vi "Lab Panel V6.00.vi"() -> ()   [LabVIEW 2017] (continued)
                            n2530 = Bundle(cluster=w4592, "amps"=w4596, "volts"=w4595, "pf"=w4594) -> (w4593:cluster{"amps":dbl, "volts":dbl, "pf":dbl})
                            n2531 = local write "ON L03-2"(w4593) -> ()
                          }
                        }
                      }
                      frame #1 {
                        n2532 = Unbundle(w4601) -> ("amps"=w4600:dbl, "volts"=w4599:dbl, "pf"=w4598:dbl)
                        n2533 = case shown="True" w4602 {
                          tunnel: w4609 -> [_ w4641]
                          tunnel: w4608 -> [_ w4648]
                          tunnel: w4607 -> [_ _]
                          tunnel: w4606 -> [_ _]
                          tunnel: w4605 -> [_ w4647]
                          tunnel: w4604 -> [_ w4646]
                          tunnel: w4603 -> [_ w4611]
                          tunnel: w4600 -> [_ w4643]
                          tunnel: w4599 -> [_ w4642]
                          tunnel: w4598 -> [_ w4640]
                          tunnel: w4597 -> [_ w4632]
                          frame False {
                          }
                          frame True {
                            n2534 = local read "TDMS LAB03-2"() -> (w4645:refnum<k34>)
                            n2535 = Build Array(w4642) -> (w4637:dbl[])
                            n2536 = Build Array(w4640) -> (w4636:dbl[])
                            n2537 = Build Array(w4647) -> (w4635:dbl[])
                            n2538 = Build Array(w4648) -> (w4634:dbl[])
                            n2539 = Build Array(w4643) -> (w4639:dbl[])
                            n2540 = Build Array(w4641) -> (w4638:dbl[])
                            n2541 = Build Array(w4646) -> (w4633:dbl[])
                            n2542 = Build Array("AMPS ON", "AMPS OFF", "VOLTS", "PF", "TEMP Live", "TEMP Neut", "CYCLE") -> (w4616:string[])
                            n2543 = Bundle By Name("Y"=w4639, "t0"=w4632) -> (w4631:waveform(dbl))  [unwired: 1 in]
                            n2544 = Bundle By Name("Y"=w4638, "t0"=w4632) -> (w4630:waveform(dbl))  [unwired: 1 in]
                            n2545 = Bundle By Name("Y"=w4637, "t0"=w4632) -> (w4629:waveform(dbl))  [unwired: 1 in]
                            n2546 = Bundle By Name("Y"=w4636, "t0"=w4632) -> (w4628:waveform(dbl))  [unwired: 1 in]
                            n2547 = Bundle By Name("Y"=w4635, "t0"=w4632) -> (w4627:waveform(dbl))  [unwired: 1 in]
                            n2548 = Bundle By Name("Y"=w4634, "t0"=w4632) -> (w4626:waveform(dbl))  [unwired: 1 in]
                            n2549 = Bundle By Name("Y"=w4633, "t0"=w4632) -> (w4625:waveform(dbl))  [unwired: 1 in]
                            n2550 = Build Array(w4631, w4630, w4629, w4628, w4627, w4626, w4625) -> (w4624:waveform(dbl)[])
                            n2551 = TDMS Write(0:w4645, 5:"TEST VALUES", 7:w4616, 9:w4624) -> (4:w4615:refnum<k34>, 6:w4614:string, 15:w4613:errorcluster)  [unwired: 2 in, 1 out]
                            n2552 = TDMS Write(0:w4615, 5:w4614, 7:"TIME", 9:w4611, 11:w4613) -> (15:w4610:errorcluster)  [unwired: 1 in, 3 out]
                            n2553 = local write "data file error"(w4610) -> ()
                          }
                        }
                      }
                    }
                  }
                }
              }
              frame #6 {
                n2554 = case shown="True" w4649 {
                  tunnel: w4653 -> [_ w4658]
                  tunnel: w4652 -> [_ w4657]
                  tunnel: w4651 -> [_ w4655]
                  tunnel: w4650 -> [_ w4654]
                  frame False {
                  }
                  frame True {
                    n2555 = local read "DISP LAB04-1"() -> (w4659:T4)
                    n2556 = local read "SIG LAB04-1"() -> (w4660:T2)
                    n2557 = local read "ON L04-1"() -> (w4656:cluster{"amps":dbl, "volts":dbl, "pf":dbl})
                    n2558 = Unbundle(w4660) -> ("AMPS"=w4666:dbl, "VOLTS"=w4664:dbl, "PF"=w4663:dbl, "Tmp Live"=w4662:dbl, "Tmp Neut"=w4665:dbl)
                    n2559 = Unbundle(w4659) -> ("CYCLE"=w4661:dbl)  [unwired: 2 out]
                    n2560 = stacked-sequence {
                      tunnel: w4666 -> [w4670 w4689]
                      tunnel: w4665 -> [_ w4688]
                      tunnel: w4664 -> [w4669 w4687]
                      tunnel: w4663 -> [w4668 w4686]
                      tunnel: w4662 -> [_ w4685]
                      tunnel: w4661 -> [_ w4684]
                      tunnel: w4658 -> [_ w4683]
                      tunnel: w4657 -> [w4671 _]
                      tunnel: w4656 -> [w4667 w4681]
                      tunnel: w4655 -> [_ w4682]
                      tunnel: w4654 -> [_ w4677]
                      frame #0 {
                        n2561 = case shown="True" w4671 {
                          tunnel: w4670 -> [_ w4676]
                          tunnel: w4669 -> [_ w4675]
                          tunnel: w4668 -> [_ w4674]
                          tunnel: w4667 -> [_ w4672]
                          frame False {
                          }
                          frame True {
                            n2562 = Bundle(cluster=w4672, "amps"=w4676, "volts"=w4675, "pf"=w4674) -> (w4673:cluster{"amps":dbl, "volts":dbl, "pf":dbl})
                            n2563 = local write "ON L04-1"(w4673) -> ()
                          }
                        }
                      }
                      frame #1 {
                        n2564 = Unbundle(w4681) -> ("amps"=w4680:dbl, "volts"=w4679:dbl, "pf"=w4678:dbl)
                        n2565 = case shown="True" w4682 {
                          tunnel: w4689 -> [_ w4721]
                          tunnel: w4688 -> [_ w4728]
                          tunnel: w4687 -> [_ _]
                          tunnel: w4686 -> [_ _]
                          tunnel: w4685 -> [_ w4727]
                          tunnel: w4684 -> [_ w4726]
                          tunnel: w4683 -> [_ w4691]
                          tunnel: w4680 -> [_ w4723]
                          tunnel: w4679 -> [_ w4722]
                          tunnel: w4678 -> [_ w4720]
                          tunnel: w4677 -> [_ w4712]
                          frame False {
                          }
                          frame True {
                            n2566 = local read "TDMS LAB04-1"() -> (w4725:refnum<k34>)
                            n2567 = Build Array(w4722) -> (w4717:dbl[])
                            n2568 = Build Array(w4720) -> (w4716:dbl[])
                            n2569 = Build Array(w4727) -> (w4715:dbl[])
                            n2570 = Build Array(w4728) -> (w4714:dbl[])
                            n2571 = Build Array(w4723) -> (w4719:dbl[])
                            n2572 = Build Array(w4721) -> (w4718:dbl[])
                            n2573 = Build Array(w4726) -> (w4713:dbl[])
                            n2574 = Build Array("AMPS ON", "AMPS OFF", "VOLTS", "PF", "TEMP Live", "TEMP Neut", "CYCLE") -> (w4696:string[])
                            n2575 = Bundle By Name("Y"=w4719, "t0"=w4712) -> (w4711:waveform(dbl))  [unwired: 1 in]
                            n2576 = Bundle By Name("Y"=w4718, "t0"=w4712) -> (w4710:waveform(dbl))  [unwired: 1 in]
                            n2577 = Bundle By Name("Y"=w4717, "t0"=w4712) -> (w4709:waveform(dbl))  [unwired: 1 in]
                            n2578 = Bundle By Name("Y"=w4716, "t0"=w4712) -> (w4708:waveform(dbl))  [unwired: 1 in]
                            n2579 = Bundle By Name("Y"=w4715, "t0"=w4712) -> (w4707:waveform(dbl))  [unwired: 1 in]
                            n2580 = Bundle By Name("Y"=w4714, "t0"=w4712) -> (w4706:waveform(dbl))  [unwired: 1 in]
                            n2581 = Bundle By Name("Y"=w4713, "t0"=w4712) -> (w4705:waveform(dbl))  [unwired: 1 in]
                            n2582 = Build Array(w4711, w4710, w4709, w4708, w4707, w4706, w4705) -> (w4704:waveform(dbl)[])
                            n2583 = TDMS Write(0:w4725, 5:"TEST VALUES", 7:w4696, 9:w4704) -> (4:w4695:refnum<k34>, 6:w4694:string, 15:w4693:errorcluster)  [unwired: 2 in, 1 out]
                            n2584 = TDMS Write(0:w4695, 5:w4694, 7:"TIME", 9:w4691, 11:w4693) -> (15:w4690:errorcluster)  [unwired: 1 in, 3 out]
                            n2585 = local write "data file error"(w4690) -> ()
                          }
                        }
                      }
                    }
                  }
                }
              }
              frame #7 {
                n2586 = case shown="True" w4729 {
                  tunnel: w4733 -> [_ w4738]
                  tunnel: w4732 -> [_ w4737]
                  tunnel: w4731 -> [_ w4735]
                  tunnel: w4730 -> [_ w4734]
                  frame False {
                  }
                  frame True {
                    n2587 = local read "DISP LAB04-2"() -> (w4739:T4)
                    n2588 = local read "SIG LAB04-2"() -> (w4740:T2)
                    n2589 = local read "ON L04-2"() -> (w4736:cluster{"amps":dbl, "volts":dbl, "pf":dbl})
                    n2590 = Unbundle(w4740) -> ("AMPS"=w4746:dbl, "VOLTS"=w4744:dbl, "PF"=w4743:dbl, "Tmp Live"=w4742:dbl, "Tmp Neut"=w4745:dbl)
                    n2591 = Unbundle(w4739) -> ("CYCLE"=w4741:dbl)  [unwired: 2 out]
                    n2592 = stacked-sequence {
                      tunnel: w4746 -> [w4750 w4769]
                      tunnel: w4745 -> [_ w4768]
                      tunnel: w4744 -> [w4749 w4767]
                      tunnel: w4743 -> [w4748 w4766]
                      tunnel: w4742 -> [_ w4765]
                      tunnel: w4741 -> [_ w4764]
                      tunnel: w4738 -> [_ w4763]
                      tunnel: w4737 -> [w4751 _]
                      tunnel: w4736 -> [w4747 w4761]
                      tunnel: w4735 -> [_ w4762]
                      tunnel: w4734 -> [_ w4757]
                      frame #0 {
                        n2593 = case shown="True" w4751 {
                          tunnel: w4750 -> [_ w4756]
                          tunnel: w4749 -> [_ w4755]
                          tunnel: w4748 -> [_ w4754]
                          tunnel: w4747 -> [_ w4752]
                          frame False {
                          }
                          frame True {
                            n2594 = Bundle(cluster=w4752, "amps"=w4756, "volts"=w4755, "pf"=w4754) -> (w4753:cluster{"amps":dbl, "volts":dbl, "pf":dbl})
                            n2595 = local write "ON L04-2"(w4753) -> ()
                          }
                        }
                      }
                      frame #1 {
                        n2596 = Unbundle(w4761) -> ("amps"=w4760:dbl, "volts"=w4759:dbl, "pf"=w4758:dbl)
                        n2597 = case shown="True" w4762 {
                          tunnel: w4769 -> [_ w4801]
                          tunnel: w4768 -> [_ w4808]
                          tunnel: w4767 -> [_ _]
                          tunnel: w4766 -> [_ _]
                          tunnel: w4765 -> [_ w4807]
                          tunnel: w4764 -> [_ w4806]
                          tunnel: w4763 -> [_ w4771]
                          tunnel: w4760 -> [_ w4803]
                          tunnel: w4759 -> [_ w4802]
                          tunnel: w4758 -> [_ w4800]
                          tunnel: w4757 -> [_ w4792]
                          frame False {
                          }
                          frame True {
                            n2598 = local read "TDMS LAB04-2"() -> (w4805:refnum<k34>)
                            n2599 = Build Array(w4802) -> (w4797:dbl[])
                            n2600 = Build Array(w4800) -> (w4796:dbl[])
                            n2601 = Build Array(w4807) -> (w4795:dbl[])
                            n2602 = Build Array(w4808) -> (w4794:dbl[])
                            n2603 = Build Array(w4803) -> (w4799:dbl[])
                            n2604 = Build Array(w4801) -> (w4798:dbl[])
                            n2605 = Build Array(w4806) -> (w4793:dbl[])
                            n2606 = Build Array("AMPS ON", "AMPS OFF", "VOLTS", "PF", "TEMP Live", "TEMP Neut", "CYCLE") -> (w4776:string[])
                            n2607 = Bundle By Name("Y"=w4799, "t0"=w4792) -> (w4791:waveform(dbl))  [unwired: 1 in]
                            n2608 = Bundle By Name("Y"=w4798, "t0"=w4792) -> (w4790:waveform(dbl))  [unwired: 1 in]
                            n2609 = Bundle By Name("Y"=w4797, "t0"=w4792) -> (w4789:waveform(dbl))  [unwired: 1 in]
                            n2610 = Bundle By Name("Y"=w4796, "t0"=w4792) -> (w4788:waveform(dbl))  [unwired: 1 in]
                            n2611 = Bundle By Name("Y"=w4795, "t0"=w4792) -> (w4787:waveform(dbl))  [unwired: 1 in]
                            n2612 = Bundle By Name("Y"=w4794, "t0"=w4792) -> (w4786:waveform(dbl))  [unwired: 1 in]
                            n2613 = Bundle By Name("Y"=w4793, "t0"=w4792) -> (w4785:waveform(dbl))  [unwired: 1 in]
                            n2614 = Build Array(w4791, w4790, w4789, w4788, w4787, w4786, w4785) -> (w4784:waveform(dbl)[])
                            n2615 = TDMS Write(0:w4805, 5:"TEST VALUES", 7:w4776, 9:w4784) -> (4:w4775:refnum<k34>, 6:w4774:string, 15:w4773:errorcluster)  [unwired: 2 in, 1 out]
                            n2616 = TDMS Write(0:w4775, 5:w4774, 7:"TIME", 9:w4771, 11:w4773) -> (15:w4770:errorcluster)  [unwired: 1 in, 3 out]
                            n2617 = local write "data file error"(w4770) -> ()
                          }
                        }
                      }
                    }
                  }
                }
              }
              frame #8 {
                n2618 = case shown="True" w4809 {
                  tunnel: w4813 -> [_ w4818]
                  tunnel: w4812 -> [_ w4817]
                  tunnel: w4811 -> [_ w4815]
                  tunnel: w4810 -> [_ w4814]
                  frame False {
                  }
                  frame True {
                    n2619 = local read "DISP LAB05-1"() -> (w4819:T4)
                    n2620 = local read "SIG LAB05-1"() -> (w4820:T2)
                    n2621 = local read "ON L05-1"() -> (w4816:cluster{"amps":dbl, "volts":dbl, "pf":dbl})
                    n2622 = Unbundle(w4820) -> ("AMPS"=w4826:dbl, "VOLTS"=w4824:dbl, "PF"=w4823:dbl, "Tmp Live"=w4822:dbl, "Tmp Neut"=w4825:dbl)
                    n2623 = Unbundle(w4819) -> ("CYCLE"=w4821:dbl)  [unwired: 2 out]
                    n2624 = stacked-sequence {
                      tunnel: w4826 -> [w4830 w4849]
                      tunnel: w4825 -> [_ w4848]
                      tunnel: w4824 -> [w4829 w4847]
                      tunnel: w4823 -> [w4828 w4846]
                      tunnel: w4822 -> [_ w4845]
                      tunnel: w4821 -> [_ w4844]
                      tunnel: w4818 -> [_ w4843]
                      tunnel: w4817 -> [w4831 _]
                      tunnel: w4816 -> [w4827 w4841]
                      tunnel: w4815 -> [_ w4842]
                      tunnel: w4814 -> [_ w4837]
                      frame #0 {
                        n2625 = case shown="True" w4831 {
                          tunnel: w4830 -> [_ w4836]
                          tunnel: w4829 -> [_ w4835]
                          tunnel: w4828 -> [_ w4834]
                          tunnel: w4827 -> [_ w4832]
                          frame False {
                          }
                          frame True {
                            n2626 = Bundle(cluster=w4832, "amps"=w4836, "volts"=w4835, "pf"=w4834) -> (w4833:cluster{"amps":dbl, "volts":dbl, "pf":dbl})
                            n2627 = local write "ON L05-1"(w4833) -> ()
                          }
                        }
                      }
                      frame #1 {
                        n2628 = Unbundle(w4841) -> ("amps"=w4840:dbl, "volts"=w4839:dbl, "pf"=w4838:dbl)
                        n2629 = case shown="True" w4842 {
                          tunnel: w4849 -> [_ w4881]
                          tunnel: w4848 -> [_ w4888]
                          tunnel: w4847 -> [_ _]
                          tunnel: w4846 -> [_ _]
                          tunnel: w4845 -> [_ w4887]
                          tunnel: w4844 -> [_ w4886]
                          tunnel: w4843 -> [_ w4851]
                          tunnel: w4840 -> [_ w4883]
                          tunnel: w4839 -> [_ w4882]
                          tunnel: w4838 -> [_ w4880]
                          tunnel: w4837 -> [_ w4872]
                          frame False {
                          }
                          frame True {
                            n2630 = local read "TDMS LAB05-1"() -> (w4885:refnum<k34>)
                            n2631 = Build Array(w4882) -> (w4877:dbl[])
                            n2632 = Build Array(w4880) -> (w4876:dbl[])
                            n2633 = Build Array(w4887) -> (w4875:dbl[])
                            n2634 = Build Array(w4888) -> (w4874:dbl[])
                            n2635 = Build Array(w4883) -> (w4879:dbl[])
                            n2636 = Build Array(w4881) -> (w4878:dbl[])
                            n2637 = Build Array(w4886) -> (w4873:dbl[])
                            n2638 = Build Array("AMPS ON", "AMPS OFF", "VOLTS", "PF", "TEMP Live", "TEMP Neut", "CYCLE") -> (w4856:string[])
                            n2639 = Bundle By Name("Y"=w4879, "t0"=w4872) -> (w4871:waveform(dbl))  [unwired: 1 in]
                            n2640 = Bundle By Name("Y"=w4878, "t0"=w4872) -> (w4870:waveform(dbl))  [unwired: 1 in]
                            n2641 = Bundle By Name("Y"=w4877, "t0"=w4872) -> (w4869:waveform(dbl))  [unwired: 1 in]
                            n2642 = Bundle By Name("Y"=w4876, "t0"=w4872) -> (w4868:waveform(dbl))  [unwired: 1 in]
                            n2643 = Bundle By Name("Y"=w4875, "t0"=w4872) -> (w4867:waveform(dbl))  [unwired: 1 in]
                            n2644 = Bundle By Name("Y"=w4874, "t0"=w4872) -> (w4866:waveform(dbl))  [unwired: 1 in]
                            n2645 = Bundle By Name("Y"=w4873, "t0"=w4872) -> (w4865:waveform(dbl))  [unwired: 1 in]
                            n2646 = Build Array(w4871, w4870, w4869, w4868, w4867, w4866, w4865) -> (w4864:waveform(dbl)[])
                            n2647 = TDMS Write(0:w4885, 5:"TEST VALUES", 7:w4856, 9:w4864) -> (4:w4855:refnum<k34>, 6:w4854:string, 15:w4853:errorcluster)  [unwired: 2 in, 1 out]
                            n2648 = TDMS Write(0:w4855, 5:w4854, 7:"TIME", 9:w4851, 11:w4853) -> (15:w4850:errorcluster)  [unwired: 1 in, 3 out]
                            n2649 = local write "data file error"(w4850) -> ()
                          }
                        }
                      }
                    }
                  }
                }
              }
              frame #9 {
                n2650 = case shown="True" w4889 {
                  tunnel: w4893 -> [_ w4898]
                  tunnel: w4892 -> [_ w4897]
                  tunnel: w4891 -> [_ w4895]
                  tunnel: w4890 -> [_ w4894]
                  frame False {
                  }
                  frame True {
                    n2651 = local read "DISP LAB05-2"() -> (w4899:T4)
                    n2652 = local read "SIG LAB05-2"() -> (w4900:T2)
                    n2653 = local read "ON L05-2"() -> (w4896:cluster{"amps":dbl, "volts":dbl, "pf":dbl})
                    n2654 = Unbundle(w4900) -> ("AMPS"=w4906:dbl, "VOLTS"=w4904:dbl, "PF"=w4903:dbl, "Tmp Live"=w4902:dbl, "Tmp Neut"=w4905:dbl)
                    n2655 = Unbundle(w4899) -> ("CYCLE"=w4901:dbl)  [unwired: 2 out]
                    n2656 = stacked-sequence {
                      tunnel: w4906 -> [w4910 w4929]
                      tunnel: w4905 -> [_ w4928]
                      tunnel: w4904 -> [w4909 w4927]
                      tunnel: w4903 -> [w4908 w4926]
                      tunnel: w4902 -> [_ w4925]
                      tunnel: w4901 -> [_ w4924]
                      tunnel: w4898 -> [_ w4923]
                      tunnel: w4897 -> [w4911 _]
                      tunnel: w4896 -> [w4907 w4921]
                      tunnel: w4895 -> [_ w4922]
                      tunnel: w4894 -> [_ w4917]
                      frame #0 {
                        n2657 = case shown="True" w4911 {
                          tunnel: w4910 -> [_ w4916]
                          tunnel: w4909 -> [_ w4915]
                          tunnel: w4908 -> [_ w4914]
                          tunnel: w4907 -> [_ w4912]
                          frame False {
                          }
                          frame True {
                            n2658 = Bundle(cluster=w4912, "amps"=w4916, "volts"=w4915, "pf"=w4914) -> (w4913:cluster{"amps":dbl, "volts":dbl, "pf":dbl})
                            n2659 = local write "ON L05-2"(w4913) -> ()
                          }
                        }
                      }
                      frame #1 {
                        n2660 = Unbundle(w4921) -> ("amps"=w4920:dbl, "volts"=w4919:dbl, "pf"=w4918:dbl)
                        n2661 = case shown="True" w4922 {
                          tunnel: w4929 -> [_ w4961]
                          tunnel: w4928 -> [_ w4968]
                          tunnel: w4927 -> [_ _]
                          tunnel: w4926 -> [_ _]
                          tunnel: w4925 -> [_ w4967]
                          tunnel: w4924 -> [_ w4966]
                          tunnel: w4923 -> [_ w4931]
                          tunnel: w4920 -> [_ w4963]
                          tunnel: w4919 -> [_ w4962]
                          tunnel: w4918 -> [_ w4960]
                          tunnel: w4917 -> [_ w4952]
                          frame False {
                          }
                          frame True {
                            n2662 = local read "TDMS LAB05-2"() -> (w4965:refnum<k34>)
                            n2663 = Build Array(w4962) -> (w4957:dbl[])
                            n2664 = Build Array(w4960) -> (w4956:dbl[])
                            n2665 = Build Array(w4967) -> (w4955:dbl[])
                            n2666 = Build Array(w4968) -> (w4954:dbl[])
                            n2667 = Build Array(w4963) -> (w4959:dbl[])
                            n2668 = Build Array(w4961) -> (w4958:dbl[])
                            n2669 = Build Array(w4966) -> (w4953:dbl[])
                            n2670 = Build Array("AMPS ON", "AMPS OFF", "VOLTS", "PF", "TEMP Live", "TEMP Neut", "CYCLE") -> (w4936:string[])
                            n2671 = Bundle By Name("Y"=w4959, "t0"=w4952) -> (w4951:waveform(dbl))  [unwired: 1 in]
                            n2672 = Bundle By Name("Y"=w4958, "t0"=w4952) -> (w4950:waveform(dbl))  [unwired: 1 in]
                            n2673 = Bundle By Name("Y"=w4957, "t0"=w4952) -> (w4949:waveform(dbl))  [unwired: 1 in]
                            n2674 = Bundle By Name("Y"=w4956, "t0"=w4952) -> (w4948:waveform(dbl))  [unwired: 1 in]
                            n2675 = Bundle By Name("Y"=w4955, "t0"=w4952) -> (w4947:waveform(dbl))  [unwired: 1 in]
                            n2676 = Bundle By Name("Y"=w4954, "t0"=w4952) -> (w4946:waveform(dbl))  [unwired: 1 in]
                            n2677 = Bundle By Name("Y"=w4953, "t0"=w4952) -> (w4945:waveform(dbl))  [unwired: 1 in]
                            n2678 = Build Array(w4951, w4950, w4949, w4948, w4947, w4946, w4945) -> (w4944:waveform(dbl)[])
                            n2679 = TDMS Write(0:w4965, 5:"TEST VALUES", 7:w4936, 9:w4944) -> (4:w4935:refnum<k34>, 6:w4934:string, 15:w4933:errorcluster)  [unwired: 2 in, 1 out]
                            n2680 = TDMS Write(0:w4935, 5:w4934, 7:"TIME", 9:w4931, 11:w4933) -> (15:w4930:errorcluster)  [unwired: 1 in, 3 out]
                            n2681 = local write "data file error"(w4930) -> ()
                          }
                        }
                      }
                    }
                  }
                }
              }
            }
          }
          frame #15 {
            # "display test values on chart"
            n2682 = local read "jig cycle"() -> (w4973:dbl)
            n2683 = local read "on loops"() -> (w4975:dbl)
            n2684 = Add(x=w4975, y=3) -> (x+y=w4972:dbl)
            n2685 = Equal?(x=w4973, y=3) -> (x = y?=w4971:bool)
            n2686 = Equal?(x=w4973, y=w4972) -> (x = y?=w4970:bool)
            n2687 = Or(x=w4971, y=w4970) -> (x .or. y?=w4969:bool)
            "graph flag" <- w4969
            n2688 = global write "Global display 3.vi" "graph flag"(w4969) -> ()
            n2689 = case shown="True" w4969 {
              frame False {
              }
              frame True {
                n2690 = local read "SIG LAB05-1"() -> (w5018:T2)
                n2691 = local read "SIG LAB04-2"() -> (w5019:T2)
                n2692 = local read "SIG LAB05-2"() -> (w5017:T2)
                n2693 = local read "SIG LAB04-1"() -> (w5020:T2)
                n2694 = local read "SIG LAB01-1"() -> (w5026:T2)
                n2695 = local read "SIG LAB03-1"() -> (w5022:T2)
                n2696 = local read "SIG LAB03-2"() -> (w5021:T2)
                n2697 = local read "SIG LAB02-2"() -> (w5023:T2)
                n2698 = local read "SIG LAB02-1"() -> (w5024:T2)
                n2699 = local read "SIG LAB01-2"() -> (w5025:T2)
                n2700 = Unbundle By Name(w5026) -> ("AMPS"=w5016:dbl, "VOLTS"=w5006:dbl, "Tmp Live"=w4996:dbl, "Tmp Neut"=w4986:dbl)
                n2701 = Unbundle(w5019) -> ("AMPS"=w5009:dbl, "VOLTS"=w4999:dbl, "Tmp Live"=w4989:dbl, "Tmp Neut"=w4979:dbl)  [unwired: 1 out]
                n2702 = Unbundle(w5018) -> ("AMPS"=w5008:dbl, "VOLTS"=w4998:dbl, "Tmp Live"=w4988:dbl, "Tmp Neut"=w4978:dbl)  [unwired: 1 out]
                n2703 = Unbundle(w5017) -> ("AMPS"=w5007:dbl, "VOLTS"=w4997:dbl, "Tmp Live"=w4987:dbl, "Tmp Neut"=w4977:dbl)  [unwired: 1 out]
                n2704 = Unbundle(w5020) -> ("AMPS"=w5010:dbl, "VOLTS"=w5000:dbl, "Tmp Live"=w4990:dbl, "Tmp Neut"=w4980:dbl)  [unwired: 1 out]
                n2705 = Unbundle(w5021) -> ("AMPS"=w5011:dbl, "VOLTS"=w5001:dbl, "Tmp Live"=w4991:dbl, "Tmp Neut"=w4981:dbl)  [unwired: 1 out]
                n2706 = Unbundle(w5022) -> ("AMPS"=w5012:dbl, "VOLTS"=w5002:dbl, "Tmp Live"=w4992:dbl, "Tmp Neut"=w4982:dbl)  [unwired: 1 out]
                n2707 = Unbundle(w5023) -> ("AMPS"=w5013:dbl, "VOLTS"=w5003:dbl, "Tmp Live"=w4993:dbl, "Tmp Neut"=w4983:dbl)  [unwired: 1 out]
                n2708 = Unbundle(w5024) -> ("AMPS"=w5014:dbl, "VOLTS"=w5004:dbl, "Tmp Live"=w4994:dbl, "Tmp Neut"=w4984:dbl)  [unwired: 1 out]
                n2709 = Unbundle(w5025) -> ("AMPS"=w5015:dbl, "VOLTS"=w5005:dbl, "Tmp Live"=w4995:dbl, "Tmp Neut"=w4985:dbl)  [unwired: 1 out]
                n2710 = stacked-sequence {
                  tunnel: w5016 -> [w5058 _ _]
                  tunnel: w5015 -> [w5057 _ _]
                  tunnel: w5014 -> [w5048 _ _]
                  tunnel: w5013 -> [w5047 _ _]
                  tunnel: w5012 -> [w5037 _ _]
                  tunnel: w5011 -> [w5036 _ _]
                  tunnel: w5010 -> [_ w5081 _]
                  tunnel: w5009 -> [_ w5080 _]
                  tunnel: w5008 -> [_ w5070 _]
                  tunnel: w5007 -> [_ w5069 _]
                  tunnel: w5006 -> [w5055 _ _]
                  tunnel: w5005 -> [w5054 _ _]
                  tunnel: w5004 -> [w5045 _ _]
                  tunnel: w5003 -> [w5044 _ _]
                  tunnel: w5002 -> [w5035 _ _]
                  tunnel: w5001 -> [w5034 _ _]
                  tunnel: w5000 -> [_ w5079 _]
                  tunnel: w4999 -> [_ w5078 _]
                  tunnel: w4998 -> [_ w5068 _]
                  tunnel: w4997 -> [_ w5067 _]
                  tunnel: w4996 -> [w5052 _ _]
                  tunnel: w4995 -> [w5050 _ _]
                  tunnel: w4994 -> [w5041 _ _]
                  tunnel: w4993 -> [w5039 _ _]
                  tunnel: w4992 -> [w5033 _ _]
                  tunnel: w4991 -> [w5031 _ _]
                  tunnel: w4990 -> [_ w5077 _]
                  tunnel: w4989 -> [_ w5075 _]
                  tunnel: w4988 -> [_ w5066 _]
                  tunnel: w4987 -> [_ w5064 _]
                  tunnel: w4986 -> [w5051 _ _]
                  tunnel: w4985 -> [w5049 _ _]
                  tunnel: w4984 -> [w5040 _ _]
                  tunnel: w4983 -> [w5038 _ _]
                  tunnel: w4982 -> [w5032 _ _]
                  tunnel: w4981 -> [w5030 _ _]
                  tunnel: w4980 -> [_ w5076 _]
                  tunnel: w4979 -> [_ w5074 _]
                  tunnel: w4978 -> [_ w5065 _]
                  tunnel: w4977 -> [_ w5063 _]
                  frame #0 {
                    n2711 = Merge Signals(w5058, w5057) -> (→"LAB01 AMPS":dynamicdata)
                    n2712 = Merge Signals(w5055, w5054) -> (→"LAB01 VOLTS":dynamicdata)
                    n2713 = Merge Signals(w5035, w5034) -> (→"LAB03 VOLTS":dynamicdata)
                    n2714 = Merge Signals(w5052, w5051, w5050, w5049) -> (→"LAB01 deg C":dynamicdata)
                    n2715 = Merge Signals(w5048, w5047) -> (→"LAB02 AMPS":dynamicdata)
                    n2716 = Merge Signals(w5041, w5040, w5039, w5038) -> (→"LAB02 deg C":dynamicdata)
                    n2717 = Merge Signals(w5033, w5032, w5031, w5030) -> (→"LAB03 deg C":dynamicdata)
                    n2718 = Merge Signals(w5045, w5044) -> (→"LAB02 VOLTS":dynamicdata)
                    n2719 = Merge Signals(w5037, w5036) -> (→"LAB03 AMPS":dynamicdata)
                  }
                  frame #1 {
                    n2720 = Merge Signals(w5068, w5067) -> (→"LAB05 VOLTS":dynamicdata)
                    n2721 = Merge Signals(w5081, w5080) -> (→"LAB04 AMPS":dynamicdata)
                    n2722 = Merge Signals(w5070, w5069) -> (→"LAB05 AMPS":dynamicdata)
                    n2723 = Merge Signals(w5066, w5065, w5064, w5063) -> (→"LAB05 deg C":dynamicdata)
                    n2724 = Merge Signals(w5077, w5076, w5075, w5074) -> (→"LAB04 deg C":dynamicdata)
                    n2725 = Merge Signals(w5079, w5078) -> (→"LAB04 VOLTS":dynamicdata)
                  }
                  frame #2 {
                    n2726 = local read "LAB05 VOLTS"() -> (w5089:dynamicdata)
                    n2727 = local read "LAB04 VOLTS"() -> (w5090:dynamicdata)
                    n2728 = local read "LAB05 AMPS"() -> (w5095:dynamicdata)
                    n2729 = local read "LAB02 VOLTS"() -> (w5092:dynamicdata)
                    n2730 = local read "LAB03 VOLTS"() -> (w5091:dynamicdata)
                    n2731 = local read "LAB01 VOLTS"() -> (w5093:dynamicdata)
                    n2732 = local read "LAB04 AMPS"() -> (w5096:dynamicdata)
                    n2733 = local read "LAB03 AMPS"() -> (w5097:dynamicdata)
                    n2734 = local read "LAB03 deg C"() -> (w5085:dynamicdata)
                    n2735 = local read "LAB02 AMPS"() -> (w5098:dynamicdata)
                    n2736 = local read "LAB04 deg C"() -> (w5084:dynamicdata)
                    n2737 = local read "LAB05 deg C"() -> (w5083:dynamicdata)
                    n2738 = local read "LAB02 deg C"() -> (w5086:dynamicdata)
                    n2739 = local read "LAB01 deg C"() -> (w5087:dynamicdata)
                    n2740 = local read "LAB01 AMPS"() -> (w5099:dynamicdata)
                    n2741 = Merge Signals(w5087, w5086, w5085, w5084, w5083) -> (w5082:dynamicdata)
                    n2742 = Merge Signals(w5099, w5098, w5097, w5096, w5095) -> (w5094:dynamicdata)
                    n2743 = Merge Signals(w5093, w5092, w5091, w5090, w5089) -> (w5088:dynamicdata)
                    n2744 = global write "Global display 3.vi" "graph volts"(w5088) -> ()
                    n2745 = global write "Global display 3.vi" "graph deg C"(w5082) -> ()
                    n2746 = global write "Global display 3.vi" "graph amps"(w5094) -> ()
                  }
                }
              }
            }
          }
          frame #16 {
            # "check for amps fail"
            # "check for cycle test & temperature rise fail conditions"
            n2747 = local read "on loops"() -> (w5127:dbl)
            n2748 = local read "jig cycle"() -> (w5124:dbl)
            n2749 = Add(x=w5127, y=5.0) -> (x+y=w5125:dbl)
            n2750 = Equal?(x=w5124, y=w5125) -> (x = y?=w5120:bool)
            n2751 = local read "jig cycle"() -> (w5129:dbl)
            n2752 = local read "TempErrors"() -> (w5100:bool[])
            n2753 = Equal?(x=w5129, y=3.0) -> (x = y?=w5122:bool)
            n2754 = local read "Fail Loops"() -> (w5101:dbl)
            n2755 = stacked-sequence {
              tunnel: w5123 -> [w5136 _ _ _ _ _ _ _ _ _]
              tunnel: w5122 -> [w5137 w5162 w5188 w5214 w5240 w5266 w5292 w5318 w5344 w5370]
              tunnel: w5121 -> [w5133 _ _ _ _ _ _ _ _ _]
              tunnel: w5120 -> [w5135 w5161 w5187 w5213 w5239 w5265 w5291 w5317 w5343 w5369]
              tunnel: w5119 -> [_ w5159 _ _ _ _ _ _ _ _]
              tunnel: w5118 -> [_ w5160 _ _ _ _ _ _ _ _]
              tunnel: w5117 -> [_ _ w5182 _ _ _ _ _ _ _]
              tunnel: w5116 -> [_ _ w5186 _ _ _ _ _ _ _]
              tunnel: w5115 -> [_ _ _ w5209 _ _ _ _ _ _]
              tunnel: w5114 -> [_ _ _ w5212 _ _ _ _ _ _]
              tunnel: w5113 -> [_ _ _ _ w5233 _ _ _ _ _]
              tunnel: w5112 -> [_ _ _ _ w5238 _ _ _ _ _]
              tunnel: w5111 -> [_ _ _ _ _ w5259 _ _ _ _]
              tunnel: w5110 -> [_ _ _ _ _ w5264 _ _ _ _]
              tunnel: w5109 -> [_ _ _ _ _ _ w5285 _ _ _]
              tunnel: w5108 -> [_ _ _ _ _ _ w5290 _ _ _]
              tunnel: w5107 -> [_ _ _ _ _ _ _ w5311 _ _]
              tunnel: w5106 -> [_ _ _ _ _ _ _ w5316 _ _]
              tunnel: w5105 -> [_ _ _ _ _ _ _ _ w5337 _]
              tunnel: w5104 -> [_ _ _ _ _ _ _ _ w5342 _]
              tunnel: w5103 -> [_ _ _ _ _ _ _ _ _ w5363]
              tunnel: w5102 -> [_ _ _ _ _ _ _ _ _ w5368]
              tunnel: w5100 -> [w5134 w5157 w5184 w5206 w5234 w5260 w5286 w5312 w5338 w5364]
              frame #0 {
                # "LAB01-1"
                n2756 = Index Array(array=w5134) -> (element=w5132:bool)  [unwired: 1 in]
                n2757 = Not(x=w5132) -> (.not. x?=w5131:bool)
                n2758 = And(x=w5131, y=w5133) -> (x .and. y?=w5130:bool)
                n2759 = case shown="True" w5130 {
                  tunnel: w5137 -> [_ w5151]
                  tunnel: w5136 -> [_ w5148]
                  tunnel: w5135 -> [_ w5147]
                  frame False {
                  }
                  frame True {
                    n2760 = local read "TEMP START LAB01-1"() -> (w5153:cluster{"TL":dbl, "TN":dbl})
                    n2761 = local read "RESULT LAB01-1"() -> (w5142:bool)
                    n2762 = local read "FAIL LAB01-1"() -> (w5145:cluster{"LO":dbl, "HI":dbl})
                    n2763 = local read "TDMS LAB01-1"() -> (w5152:refnum<k34>)
                    n2764 = local read "SET LAB01-1"() -> (w5149:T5)
                    n2765 = local read "DISP LAB01-1"() -> (w5150:T4)
                    n2766 = local read "SIG LAB01-1"() -> (w5154:T2)
                    n2767 = Bundle("FAIL LAB01-1"=w5145, "SIG LAB01-1"=w5154, "TEMP START LAB01-1"=w5153, "DISP LAB01-1"=w5150, "SET LAB01-1"=w5149, "TDMS LAB01-1"=w5152) -> (w5139:T39)  [unwired: 1 in]
                    n2768 = call "sub vi - cycle&temp fail v7.vi"("Amps Lo?"=w5151, "Input Cluster"=w5139, "SELECT"=w5148, "Amps Hi?"=w5147, "Result In"=w5142, "Panel"=u64 1) -> ("(FAIL) out"=w5144:cluster{"FAIL LO":dbl, "FAIL HI":dbl}, "(DISP) out"=w5140:T40, "T-RISE"=w5141:cluster{"T-RISE (L)":dbl, "T-RISE (N)":dbl}, "Result Out"=w5143:bool, "file error"=w5146:errorcluster)  [unwired: 9 in]
                    n2769 = local write "TEMP RISE LAB01-1"(w5141) -> ()
                    n2770 = local write "FAIL LAB01-1"(w5144) -> ()
                    n2771 = local write "DISP LAB01-1"(w5140) -> ()
                    n2772 = local write "RESULT LAB01-1"(w5143) -> ()
                    n2773 = local write "data file error"(w5146) -> ()
                  }
                }
              }
              frame #1 {
                # "LAB01-2"
                n2774 = Index Array(array=w5157) -> (element=w5158:bool)  [unwired: 1 in]
                n2775 = Not(x=w5158) -> (.not. x?=w5156:bool)
                n2776 = And(x=w5156, y=w5159) -> (x .and. y?=w5155:bool)
                n2777 = case shown="True" w5155 {
                  tunnel: w5162 -> [_ w5176]
                  tunnel: w5160 -> [_ w5173]
                  tunnel: w5161 -> [_ w5172]
                  frame False {
                  }
                  frame True {
                    n2778 = local read "TEMP START LAB01-2"() -> (w5178:cluster{"TL":dbl, "TN":dbl})
                    n2779 = local read "TDMS LAB01-2"() -> (w5177:refnum<k34>)
                    n2780 = local read "SET LAB01-2"() -> (w5174:T5)
                    n2781 = local read "DISP LAB01-2"() -> (w5175:T4)
                    n2782 = local read "FAIL LAB01-2"() -> (w5169:cluster{"LO":dbl, "HI":dbl})
                    n2783 = local read "RESULT LAB01-2"() -> (w5166:bool)
                    n2784 = local read "SIG LAB01-2"() -> (w5179:T2)
                    n2785 = Bundle("FAIL LAB01-2"=w5169, "SIG LAB01-2"=w5179, "TEMP START LAB01-2"=w5178, "DISP LAB01-2"=w5175, "SET LAB01-2"=w5174, "TDMS LAB01-2"=w5177) -> (w5164:T41)  [unwired: 1 in]
                    n2786 = call "sub vi - cycle&temp fail v7.vi"("Amps Lo?"=w5176, "Input Cluster"=w5164, "SELECT"=w5173, "Amps Hi?"=w5172, "Result In"=w5166, "Panel"=u64 2) -> ("(FAIL) out"=w5168:cluster{"FAIL LO":dbl, "FAIL HI":dbl}, "(DISP) out"=w5171:T40, "T-RISE"=w5165:cluster{"T-RISE (L)":dbl, "T-RISE (N)":dbl}, "Result Out"=w5167:bool, "file error"=w5170:errorcluster)  [unwired: 9 in]
                    n2787 = local write "TEMP RISE LAB01-2"(w5165) -> ()
                    n2788 = local write "FAIL LAB01-2"(w5168) -> ()
                    n2789 = local write "DISP LAB01-2"(w5171) -> ()
                    n2790 = local write "RESULT LAB01-2"(w5167) -> ()
                    n2791 = local write "data file error"(w5170) -> ()
                  }
                }
              }
              frame #2 {
                # "LAB02-1"
                n2792 = Index Array(array=w5184, index=1) -> (element=w5185:bool)
                n2793 = Not(x=w5185) -> (.not. x?=w5181:bool)
                n2794 = And(x=w5181, y=w5182) -> (x .and. y?=w5180:bool)
                n2795 = case shown="True" w5180 {
                  tunnel: w5188 -> [_ w5202]
                  tunnel: w5186 -> [_ w5199]
                  tunnel: w5187 -> [_ w5198]
                  frame False {
                  }
                  frame True {
                    n2796 = local read "TEMP START LAB02-1"() -> (w5204:cluster{"TL":dbl, "TN":dbl})
                    n2797 = local read "FAIL LAB02-1"() -> (w5195:cluster{"LO":dbl, "HI":dbl})
                    n2798 = local read "TDMS LAB02-1"() -> (w5203:refnum<k34>)
                    n2799 = local read "SIG LAB02-1"() -> (w5205:T2)
                    n2800 = local read "DISP LAB02-1"() -> (w5201:T4)
                    n2801 = local read "SET LAB02-1"() -> (w5200:T5)
                    n2802 = local read "RESULT LAB02-1"() -> (w5192:bool)
                    n2803 = Bundle("FAIL LAB02-1"=w5195, "SIG LAB02-1"=w5205, "TEMP START LAB02-1"=w5204, "DISP LAB02-1"=w5201, "SET LAB02-1"=w5200, "TDMS LAB02-1"=w5203) -> (w5190:T42)  [unwired: 1 in]
                    n2804 = call "sub vi - cycle&temp fail v7.vi"("Amps Lo?"=w5202, "Input Cluster"=w5190, "SELECT"=w5199, "Amps Hi?"=w5198, "Result In"=w5192, "Panel"=u64 3) -> ("(FAIL) out"=w5194:cluster{"FAIL LO":dbl, "FAIL HI":dbl}, "(DISP) out"=w5197:T40, "T-RISE"=w5191:cluster{"T-RISE (L)":dbl, "T-RISE (N)":dbl}, "Result Out"=w5193:bool, "file error"=w5196:errorcluster)  [unwired: 9 in]
                    n2805 = local write "DISP LAB02-1"(w5197) -> ()
                    n2806 = local write "data file error"(w5196) -> ()
                    n2807 = local write "TEMP RISE LAB02-1"(w5191) -> ()
                    n2808 = local write "RESULT LAB02-1"(w5193) -> ()
                    n2809 = local write "FAIL LAB02-1"(w5194) -> ()
                  }
                }
              }
              frame #3 {
                # "LAB02-2"
                n2810 = Index Array(array=w5206, index=1) -> (element=w5208:bool)
                n2811 = Not(x=w5208) -> (.not. x?=w5210:bool)
                n2812 = And(x=w5210, y=w5209) -> (x .and. y?=w5207:bool)
                n2813 = case shown="True" w5207 {
                  tunnel: w5214 -> [_ w5228]
                  tunnel: w5212 -> [_ w5225]
                  tunnel: w5213 -> [_ w5224]
                  frame False {
                  }
                  frame True {
                    n2814 = local read "TEMP START LAB02-2"() -> (w5230:cluster{"TL":dbl, "TN":dbl})
                    n2815 = local read "FAIL LAB02-2"() -> (w5221:cluster{"LO":dbl, "HI":dbl})
                    n2816 = local read "TDMS LAB02-2"() -> (w5229:refnum<k34>)
                    n2817 = local read "SET LAB02-2"() -> (w5226:T5)
                    n2818 = local read "DISP LAB02-2"() -> (w5227:T4)
                    n2819 = local read "SIG LAB02-2"() -> (w5231:T2)
                    n2820 = local read "RESULT LAB02-2"() -> (w5218:bool)
                    n2821 = Bundle("FAIL LAB02-2"=w5221, "SIG LAB02-2"=w5231, "TEMP START LAB02-2"=w5230, "DISP LAB02-2"=w5227, "SET LAB02-2"=w5226, "TDMS LAB02-2"=w5229) -> (w5216:T43)  [unwired: 1 in]
                    n2822 = call "sub vi - cycle&temp fail v7.vi"("Amps Lo?"=w5228, "Input Cluster"=w5216, "SELECT"=w5225, "Amps Hi?"=w5224, "Result In"=w5218, "Panel"=u64 4) -> ("(FAIL) out"=w5220:cluster{"FAIL LO":dbl, "FAIL HI":dbl}, "(DISP) out"=w5223:T40, "T-RISE"=w5217:cluster{"T-RISE (L)":dbl, "T-RISE (N)":dbl}, "Result Out"=w5219:bool, "file error"=w5222:errorcluster)  [unwired: 9 in]
                    n2823 = local write "TEMP RISE LAB02-2"(w5217) -> ()
                    n2824 = local write "FAIL LAB02-2"(w5220) -> ()
                    n2825 = local write "DISP LAB02-2"(w5223) -> ()
                    n2826 = local write "RESULT LAB02-2"(w5219) -> ()
                    n2827 = local write "data file error"(w5222) -> ()
                  }
                }
              }
              frame #4 {
                # "LAB03-1"
                n2828 = Index Array(array=w5234, index=2) -> (element=w5237:bool)
                n2829 = Not(x=w5237) -> (.not. x?=w5235:bool)
                n2830 = And(x=w5235, y=w5233) -> (x .and. y?=w5232:bool)
                n2831 = case shown="True" w5232 {
                  tunnel: w5240 -> [_ w5254]
                  tunnel: w5238 -> [_ w5251]
                  tunnel: w5239 -> [_ w5250]
                  frame False {
                  }
                  frame True {
                    n2832 = local read "TEMP START LAB03-1"() -> (w5256:cluster{"TL":dbl, "TN":dbl})
                    n2833 = local read "FAIL LAB03-1"() -> (w5247:cluster{"LO":dbl, "HI":dbl})
                    n2834 = local read "TDMS LAB03-1"() -> (w5255:refnum<k34>)
                    n2835 = local read "SET LAB03-1"() -> (w5252:T5)
                    n2836 = local read "DISP LAB03-1"() -> (w5253:T4)
                    n2837 = local read "SIG LAB03-1"() -> (w5257:T2)
                    n2838 = local read "RESULT LAB03-1"() -> (w5244:bool)
                    n2839 = Bundle("FAIL LAB03-1"=w5247, "SIG LAB03-1"=w5257, "TEMP START LAB03-1"=w5256, "DISP LAB03-1"=w5253, "SET LAB03-1"=w5252, "TDMS LAB03-1"=w5255) -> (w5242:T44)  [unwired: 1 in]
                    n2840 = call "sub vi - cycle&temp fail v7.vi"("Amps Lo?"=w5254, "Input Cluster"=w5242, "SELECT"=w5251, "Amps Hi?"=w5250, "Result In"=w5244, "Panel"=u64 5) -> ("(FAIL) out"=w5246:cluster{"FAIL LO":dbl, "FAIL HI":dbl}, "(DISP) out"=w5249:T40, "T-RISE"=w5243:cluster{"T-RISE (L)":dbl, "T-RISE (N)":dbl}, "Result Out"=w5245:bool, "file error"=w5248:errorcluster)  [unwired: 9 in]
                    n2841 = local write "TEMP RISE LAB03-1"(w5243) -> ()
                    n2842 = local write "FAIL LAB03-1"(w5246) -> ()
                    n2843 = local write "DISP LAB03-1"(w5249) -> ()
                    n2844 = local write "RESULT LAB03-1"(w5245) -> ()
                    n2845 = local write "data file error"(w5248) -> ()
                  }
                }
              }
              frame #5 {
                # "LAB03-2"
                n2846 = Index Array(array=w5260, index=2) -> (element=w5263:bool)
                n2847 = Not(x=w5263) -> (.not. x?=w5261:bool)
                n2848 = And(x=w5261, y=w5259) -> (x .and. y?=w5258:bool)
                n2849 = case shown="True" w5258 {
                  tunnel: w5266 -> [_ w5280]
                  tunnel: w5264 -> [_ w5277]
                  tunnel: w5265 -> [_ w5276]
                  frame False {
                  }
                  frame True {
                    n2850 = local read "TEMP START LAB03-2"() -> (w5282:cluster{"TL":dbl, "TN":dbl})
                    n2851 = local read "FAIL LAB03-2"() -> (w5273:cluster{"LO":dbl, "HI":dbl})
                    n2852 = local read "TDMS LAB03-2"() -> (w5281:refnum<k34>)
                    n2853 = local read "SET LAB03-2"() -> (w5278:T5)
                    n2854 = local read "DISP LAB03-2"() -> (w5279:T4)
                    n2855 = local read "RESULT LAB03-2"() -> (w5270:bool)
                    n2856 = local read "SIG LAB03-2"() -> (w5283:T2)
                    n2857 = Bundle("FAIL LAB03-2"=w5273, "SIG LAB03-2"=w5283, "TEMP START LAB03-2"=w5282, "DISP LAB03-2"=w5279, "SET LAB03-2"=w5278, "TDMS LAB03-2"=w5281) -> (w5268:T45)  [unwired: 1 in]
                    n2858 = call "sub vi - cycle&temp fail v7.vi"("Amps Lo?"=w5280, "Input Cluster"=w5268, "SELECT"=w5277, "Amps Hi?"=w5276, "Result In"=w5270, "Panel"=u64 6) -> ("(FAIL) out"=w5272:cluster{"FAIL LO":dbl, "FAIL HI":dbl}, "(DISP) out"=w5275:T40, "T-RISE"=w5269:cluster{"T-RISE (L)":dbl, "T-RISE (N)":dbl}, "Result Out"=w5271:bool, "file error"=w5274:errorcluster)  [unwired: 9 in]
                    n2859 = local write "FAIL LAB03-2"(w5272) -> ()
                    n2860 = local write "TEMP RISE LAB03-2"(w5269) -> ()
                    n2861 = local write "DISP LAB03-2"(w5275) -> ()
                    n2862 = local write "RESULT LAB03-2"(w5271) -> ()
                    n2863 = local write "data file error"(w5274) -> ()
                  }
                }
              }
              frame #6 {
                # "LAB04-1"
                n2864 = Index Array(array=w5286, index=3) -> (element=w5289:bool)
                n2865 = Not(x=w5289) -> (.not. x?=w5287:bool)
                n2866 = And(x=w5287, y=w5285) -> (x .and. y?=w5284:bool)
                n2867 = case shown="True" w5284 {
                  tunnel: w5292 -> [_ w5306]
                  tunnel: w5290 -> [_ w5303]
                  tunnel: w5291 -> [_ w5302]
                  frame False {
                  }
                  frame True {
                    n2868 = local read "TEMP START LAB04-1"() -> (w5308:cluster{"TL":dbl, "TN":dbl})
                    n2869 = local read "FAIL LAB04-1"() -> (w5299:cluster{"LO":dbl, "HI":dbl})
                    n2870 = local read "TDMS LAB04-1"() -> (w5307:refnum<k34>)
                    n2871 = local read "SET LAB04-1"() -> (w5304:T5)
                    n2872 = local read "DISP LAB04-1"() -> (w5305:T4)
                    n2873 = local read "SIG LAB04-1"() -> (w5309:T2)
                    n2874 = local read "RESULT LAB04-1"() -> (w5296:bool)
                    n2875 = Bundle("FAIL LAB04-1"=w5299, "SIG LAB04-1"=w5309, "TEMP START LAB04-1"=w5308, "DISP LAB04-1"=w5305, "SET LAB04-1"=w5304, "TDMS LAB04-1"=w5307) -> (w5294:T46)  [unwired: 1 in]
                    n2876 = call "sub vi - cycle&temp fail v7.vi"("Amps Lo?"=w5306, "Input Cluster"=w5294, "SELECT"=w5303, "Amps Hi?"=w5302, "Result In"=w5296, "Panel"=u64 7) -> ("(FAIL) out"=w5298:cluster{"FAIL LO":dbl, "FAIL HI":dbl}, "(DISP) out"=w5301:T40, "T-RISE"=w5295:cluster{"T-RISE (L)":dbl, "T-RISE (N)":dbl}, "Result Out"=w5297:bool, "file error"=w5300:errorcluster)  [unwired: 9 in]
                    n2877 = local write "TEMP RISE LAB04-1"(w5295) -> ()
                    n2878 = local write "FAIL LAB04-1"(w5298) -> ()
                    n2879 = local write "DISP LAB04-1"(w5301) -> ()
                    n2880 = local write "RESULT LAB04-1"(w5297) -> ()
                    n2881 = local write "data file error"(w5300) -> ()
                  }
                }
              }
              frame #7 {
                # "LAB04-2"
                n2882 = Index Array(array=w5312, index=3) -> (element=w5315:bool)
                n2883 = Not(x=w5315) -> (.not. x?=w5313:bool)
                n2884 = And(x=w5313, y=w5311) -> (x .and. y?=w5310:bool)
                n2885 = case shown="True" w5310 {
                  tunnel: w5318 -> [_ w5332]
                  tunnel: w5316 -> [_ w5329]
                  tunnel: w5317 -> [_ w5328]
                  frame False {
                  }
                  frame True {
                    n2886 = local read "TEMP START LAB04-2"() -> (w5334:cluster{"TL":dbl, "TN":dbl})
                    n2887 = local read "FAIL LAB04-2"() -> (w5325:cluster{"LO":dbl, "HI":dbl})
                    n2888 = local read "TDMS LAB04-2"() -> (w5333:refnum<k34>)
                    n2889 = local read "SET LAB04-2"() -> (w5330:T5)
                    n2890 = local read "DISP LAB04-2"() -> (w5331:T4)
